vi "Agilent Ref Type Conversion.vi"(7 "Agilent Ref":u8) -> (4 "VISA resource name":refnum<visa-resource-name>)   [LabVIEW 2012]
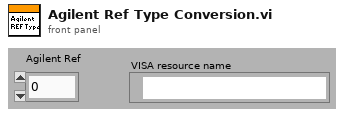
[diagram p1: front panel]
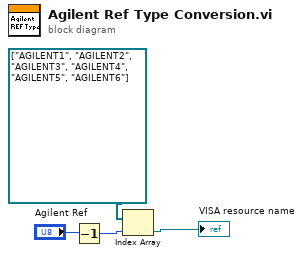
[diagram p0: block diagram]
diagram:
  n1 = Decrement(x="Agilent Ref") -> (x-1=w3:u8)
  n2 = Index Array(array=refnum<visa-resource-name>[] ["AGILENT1", "AGILENT2", "AGILENT3", "AGILENT4", "AGILENT5", "AGILENT6"] ("Array"), index=w3) -> (element=→"VISA resource name":refnum<visa-resource-name>)
